vi "Connect.vi"(6 "Timeout (60000 ms)":i32=60000, 8 "Error In":errorcluster, 10 "Address":string, 11 "Session In":refnum<class "Session.lvclass">) -> (0 "Error Out":errorcluster, 3 "Sesssion Out":refnum<class "Session.lvclass">)   [LabVIEW 2018, in "Toolkit.lvlib" / "Session.lvclass"]
doc: "Connects a sesssion to a remote SSH server. This is typically called immediately after creating the session, and this must be called BEFORE authenticating a user with the remote SSH server."
uses:
  Session.lvclass
  Session.lvclass/Session.ctl
  SSH/SSH.lvclass/SSH.ctl
  Toolkit.lvlib
  SSH/SSH.lvclass
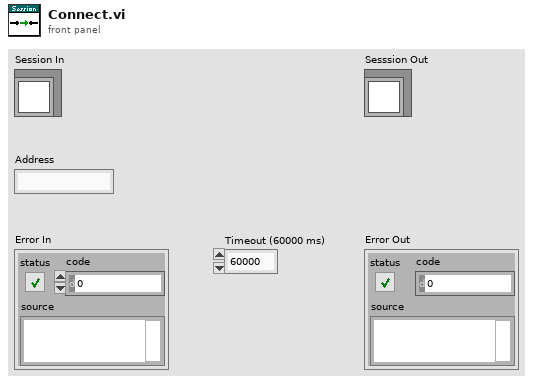
[diagram p1: front panel]
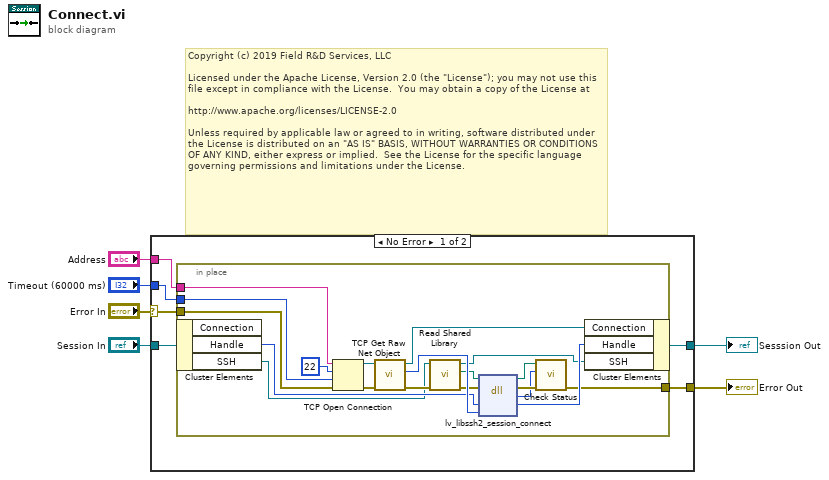
[diagram p0: block diagram]
diagram:
  # "Copyright (c) 2019 Field R&D Services, LLC\n\nLicensed under the Apache License, Version 2.0 (the \"License\"); you may not use this file except in compliance with the License.  You may obtain a copy of the License at\n\nhttp://www.apache.org/licenses/LICENSE-2.0\n\nUnless required by applicable law or agreed to in writing, software distributed under the License is distributed on an \"AS IS\" BASIS, WITHOUT WARRANTIES OR CONDITIONS OF ANY KIND, either express or implied.  See the License for the specific language governing permissions and limitations under the License."
  n1 = case shown="No Error" "Error In" {
    selector: "Error In" -> [w10 w33]
    tunnel: "Address" -> [w12 _]
    tunnel: [w11 w33] -> w4
    tunnel: "Session In" -> [w9 w32]
    tunnel: [w8 w32] -> w2
    tunnel: "Timeout (60000 ms)" -> [w7 _]
    frame No Error {
      n2 = in-place {
        in-place-border: w12 -> [w30]
        in-place-border: [w19] -> w11
        in-place-border: w10 -> [w29]
        in-place-border: w7 -> [w13]
        n3 = in-place-cluster #1(w9) -> ("Handle"=w23:u64, "SSH"=w16:refnum<class "SSH.lvclass">)  [unwired: 1 out]
        n4 = TCP Open Connection(address=w30, remote port or service name=u16 22, timeout ms (60000)=w13, error in (no error)=w29) -> (connection ID=w27:refnum<k5>, error out=w28:errorcluster)  [unwired: 1 in]
        n5 = call <vilib>:"TCP Get Raw Net Object.vi"("error in (no error)"=w28, "connection ID"=w27) -> ("error out"=w26:errorcluster, "raw net object"=w25:u64, "connection ID out"=w24:refnum<k5>)  [unwired: 7 in]
        n6 = call "Read Shared Library.vi"("Error In"=w26, "SSH In"=w16) -> ("Error Out"=w17:errorcluster, "libssh2lv Shared Library"=w14:path, "SSH Out"=w15:refnum<class "SSH.lvclass">)  [unwired: 7 in]
        n7 = dll-call lib="libssh2lv.*" fn="lv_libssh2_session_connect"(path in=w14, error in=w17, "session"=w23, "socket"=w25) -> (path out=w20:path, error out=w21:errorcluster, "result"=w18:i32, "session"=w22:u64)  [unwired: 2 in]
        n8 = call "Check Status.vi"("Error In"=w21, "Status"=w18, "libssh2lv Shared Library In"=w20) -> ("Error Out"=w19:errorcluster)  [unwired: 7 in, 1 out]
        n9 = in-place-cluster #1("Connection"=w24, "Handle"=w22, "SSH"=w15) -> (w8:refnum<class "Session.lvclass">)
      }
    }
    frame Error {
    }
  }
  "Sesssion Out" <- w2
  "Error Out" <- w4
